vi "ReadParams.vi"(11 "error in (no error)":errorcluster) -> (2 "元素":dbl, 3 "元素 2":dbl format="%#_6f", 4 "元素 3":dbl, 6 "元素 4":dbl, 8 "元素 5":dbl, 10 "元素 6":dbl, 13 "元素 7":dbl, 14 "元素 8":dbl, 15 "error out":errorcluster)   [LabVIEW 2014]
uses:
  <vilib>/addons/database/Connection.llb/DB Tools Open Connec (String).vi
  <vilib>/addons/database/Connection.llb/Conn Execute.vi
  <vilib>/addons/database/Recordset.llb/Rec Fetch Recordset Data (R).vi
  <vilib>/addons/database/Recordset.llb/Rec Destroy - Connection.vi
  <vilib>/addons/database/_DB Variant To Data/Database Variant To Data.xnode
  <vilib>/addons/database/NI_Database_API.lvlib
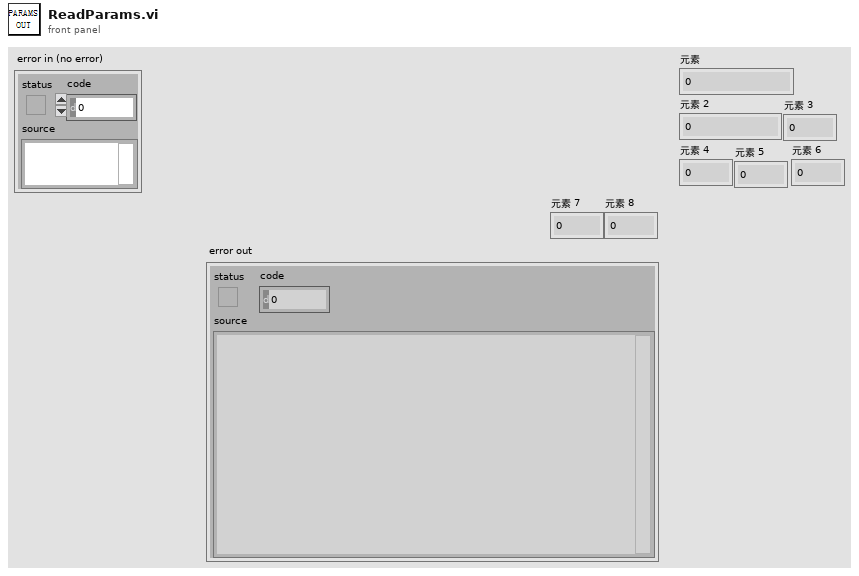
[diagram p1: front panel]
types:
  T1 = typedef "NI_Database_API.lvlib/Conn ObjectReference.ctl" = refnum<k1>
  T2 = typedef "NI_Database_API.lvlib/Rec ObjectReference.ctl" = refnum<k1>
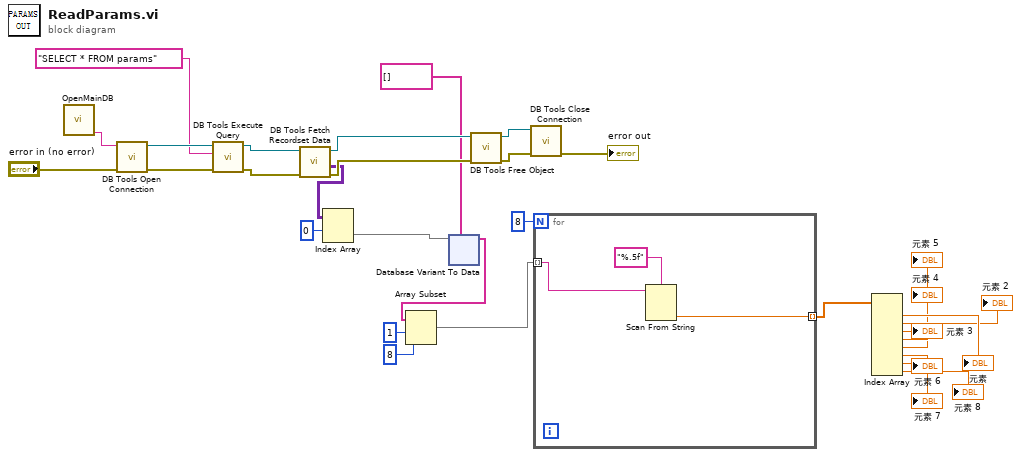
[diagram p0: block diagram]
diagram:
  n1 = call "OpenMainDB.vi"() -> ("头信息"=w30:string)  [unwired: 11 in]
  n2 = call-poly <vilib>:"DB Tools Open Connection.vi"("error in (no error)"="error in (no error)", "connection information"=w30) -> ("error out"=w26:errorcluster, "connection reference"=w27:T1)  [unwired: 6 in]
  n3 = call-poly <vilib>:"DB Tools Execute Query.vi"("error in (no error)"=w26, "SQL query"="SELECT * FROM params", "connection reference"=w27) -> ("error out"=w25:errorcluster, "recordset reference"=w28:T2)  [unwired: 5 in]
  n4 = call-poly <vilib>:"DB Tools Fetch Recordset Data.vi"("error in (no error)"=w25, "recordset reference"=w28) -> ("error out"=w22:errorcluster, "recordset data"=w18:variant[][], "recordset reference out"=w23:T2)  [unwired: 3 in]
  n5 = Index Array(array=w18, index (row)=0 ("索引 (行)")) -> (element=w16:variant[])  [unwired: 1 in]
  n6 = xnode "Database Variant To Data"("database variant"=w16, "type"=string[] []) -> ("data"=w10:string[])  [unwired: 1 in, 1 out]
  n7 = Array Subset(array=w10, index=1 ("索引"), length=8 ("长度")) -> (w7:string[])
  n8 = call-poly <vilib>:"DB Tools Free Object.vi"("error in (no error)"=w22, "recordset reference"=w23) -> ("error out"=w20:errorcluster, "connection reference"=w21:T1)  [unwired: 8 in]
  n9 = call <vilib>:"DB Tools Close Connection.vi"("error in (no error)"=w20, "connection reference"=w21) -> ("error out"=→"error out":errorcluster)  [unwired: 5 in]
  n10 = for {
    N: 8 -> [_]
    tunnel: w7 -> [w33] mode=indexing
    tunnel: [w31] -> w13 mode=indexing
    n11 = Scan From String(format string="%.5f" ("格式字符串"), input string=w33) -> (output 1=w31:dbl)  [unwired: 3 in, 3 out]
  }
  n12 = Index Array(array=w13) -> (element #1=→"元素":dbl, element #2=→"元素 2":dbl, element #3=→"元素 3":dbl, element #4=→"元素 4":dbl, element #5=→"元素 5":dbl, element #6=→"元素 6":dbl, element #7=→"元素 7":dbl, element #8=→"元素 8":dbl)  [unwired: 8 in]
